vi "CtrlTreeOpenVI.vi"(8 "VIs":map{string, string}(c390), 9 "Apps":map{string, string}(c390), 10 "Tag":string, 11 "ControlTree in":refnum<vi>) -> (0 "error out":errorcluster, 1 "Newly Opened":bool, 2 "VI ref":refnum<vi>)   [LabVIEW 2020]
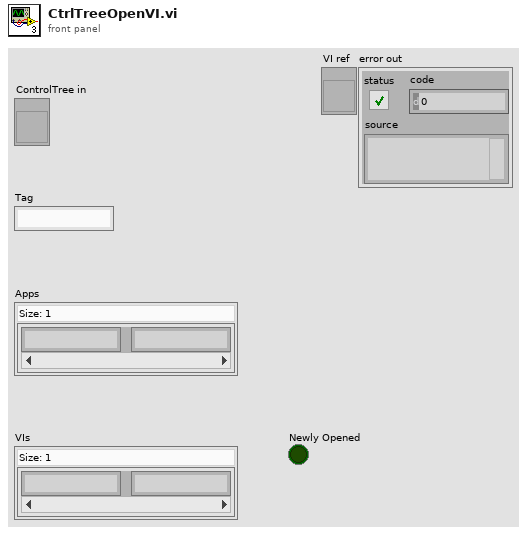
[diagram p1: front panel]
types:
  T1 = cluster{"string array[0]":string, "string array[1]":string, "string array[2]":string, "string array[3]":string}
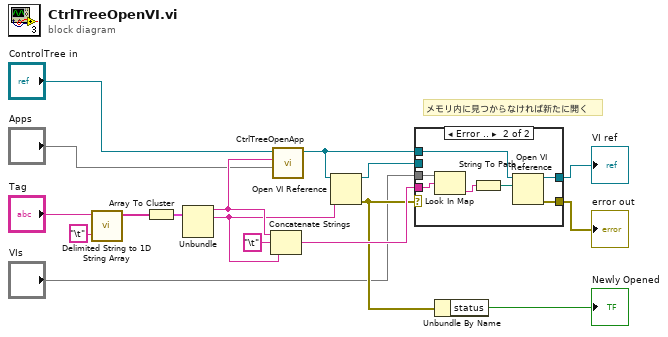
[diagram p0: block diagram]
diagram:
  # "メモリ内に見つからなければ新たに開く"
  n1 = call <vilib>:"Delimited String to 1D String Array.vi"("delimiter"="\t", "delimited string"="Tag") -> ("string array"=w16:string[])  [unwired: 9 in]
  n2 = Array To Cluster(array=w16) -> (cluster=w17:T1)
  n3 = Unbundle(w17) -> ("string array[0]"=w7:string, "string array[1]"=w6:string)  [unwired: 2 out]
  n4 = Concatenate Strings(w7, "\t" ("string"), w6) -> (w5:string)
  n5 = call "CtrlTreeOpenApp.vi"("AppPaths"="Apps", "AppName"=w7, "TreeControl in"="ControlTree in") -> ("Application out"=w9:refnum<vi>)  [unwired: 8 in]
  n6 = Open VI Reference(application reference (local)=w9, vi path=w6) -> (vi reference=w12:refnum<vi>, error out=w4:errorcluster)  [unwired: 4 in]
  n7 = case shown="Error .." w4 {
    selector: w4 -> [w18 _]
    tunnel: w12 -> [w19 _]
    tunnel: [w19 w21] -> w11
    tunnel: [w18 w20] -> w10
    tunnel: w9 -> [_ w26]
    tunnel: "VIs" -> [_ w24]
    tunnel: w5 -> [_ w25]
    frame No Error {
    }
    frame Error {
      n8 = Look In Map(map=w24, key=w25) -> (value=w23:string)  [unwired: 1 in, 1 out]
      n9 = String To Path(string=w23) -> (path=w22:path)
      n10 = Open VI Reference(application reference (local)=w26, vi path=w22) -> (vi reference=w21:refnum<vi>, error out=w20:errorcluster)  [unwired: 4 in]
    }
  }
  "VI ref" <- w11
  "error out" <- w10
  n11 = Unbundle By Name(w4) -> ("status"=→"Newly Opened":bool)
